vi "WriteToErrorLog.vi"(8 "error in":errorcluster, 9 "ErrorState(Set)":T2, 10 "Class":T1, 11 "source":string) -> (0 "error out":errorcluster)   [LabVIEW 2018]
uses:
  <vilib>/NI_Real-Time Target Support.lvlib
  Public Controls/ErrorState.ctl
  Public Controls/ClassList.ctl
panel:
  out "LastError":timestamp
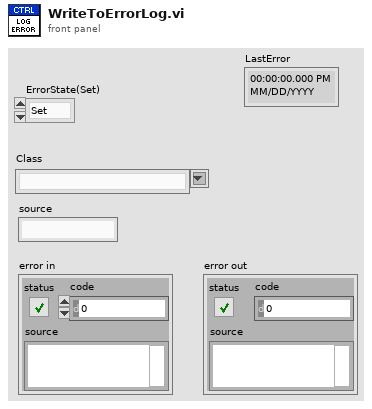
[diagram p1: front panel]
types:
  T1 = typedef "Controller.lvclass/ClassList.ctl" = string
  T2 = typedef "ErrorState.ctl" = enum16{"Set", "Get"}
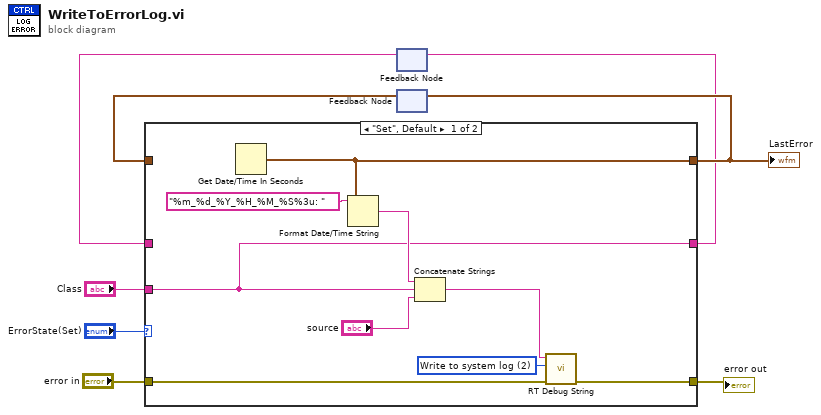
[diagram p0: block diagram]
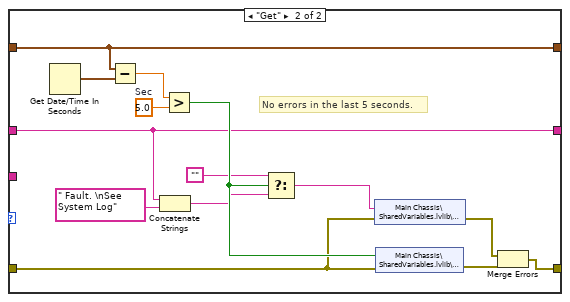
[diagram p2: hidden frame]
diagram:
  n1 = feedback #1() -> (w1:T1)  [unwired: 1 in]
  n2 = feedback #2() -> (w4:timestamp)  [unwired: 1 in]
  n3 = case shown="\"Set\", Default" "ErrorState(Set)" {
    tunnel: [w16 w18] -> w8
    tunnel: "error in" -> [w15 w21]
    tunnel: [w10 w31] -> w5
    tunnel: w4 -> [_ w31]
    tunnel: "Class" -> [w9 _]
    tunnel: [w9 w24] -> w2
    tunnel: w1 -> [_ w24]
    frame "Set", Default {
      w17 = u16 2 items=["Write to serial", "Write to monitor", "Write to system log"] ("Interface")
      n4 = Get Date/Time In Seconds() -> (seconds since 1Jan1904=w10:timestamp)
      n5 = Format Date/Time String(time format string (%c)="%m_%d_%Y_%H_%M_%S%3u: " ("format string"), seconds (now)=w10) -> (date/time string=w11:string)  [unwired: 1 in]
      n6 = Concatenate Strings(w11, w9, "source") -> (w14:string)
      n7 = call <vilib>:"RT Debug String.vi"("error in (no error)"=w15, "Interface"=w17, "String to write"=w14) -> ("error out"=w16:errorcluster)  [unwired: 8 in]
    }
    frame "Get" {
      w28 = 5.0  # Sec
      # "No errors in the last 5 seconds."
      n8 = Get Date/Time In Seconds() -> (seconds since 1Jan1904=w30:timestamp)
      n9 = Subtract(x=w31, y=w30) -> (x-y=w29:dbl)
      n10 = Concatenate Strings(w24, " Fault. \nSee System Log" ("string")) -> (w23:string)
      n11 = Greater?(x=w29, y=w28) -> (0:w26:bool)
      n12 = Select(t="", s=w26, f=w23) -> (s? t:f=w22:string)
      n13 = shared-variable "Main Chassis\\SharedVariables.lvlib\\RTStatus"(w22, error in=w21) -> (error out=w20:errorcluster)
      n14 = shared-variable "Main Chassis\\SharedVariables.lvlib\\RTGood"(w26, error in=w21) -> (error out=w19:errorcluster)
      n15 = Merge Errors(w20, w19) -> (w18:errorcluster)
    }
  }
  "error out" <- w8
  "LastError" <- w5
  n16 = feedback-in #1(w2) -> ()
  n17 = feedback-in #2(w5) -> ()
